vi "扫频仪设计.vi"() -> ()   [LabVIEW 2018]
uses:
  <vilib>/Analysis/3filter.llb/Filter Structure Type.ctl
  <vilib>/measure/macond.llb/IIR Filter for N Chan.vi
  <vilib>/measure/NI_MAPro.lvlib
  <vilib>/Analysis/NI_AALBase.lvlib
panel:
  in  "停止":bool
  out "数值 2":dbl
  out "数值":dbl
  out "波形图":cluster{"频率间隔/kHz":dbl, "频率间隔/kHz":dbl, dbl[]}(graph)
  in  "IIR filter specifications":T1={"Topology"=enum."Butterworth", "Type"=enum."Lowpass", "Order"=1, "Lower Fc"=100.0, "Upper Fc"=200.0, "PB Ripple"=1.0, "SB Attenuation"=60.0} caption="IIR滤波器规范" {"PB Ripple" format="%0.2f"; "SB Attenuation" format="%0.2f"; "Lower Fc" format="%0.2p"; "Upper Fc" format="%0.2p"}
  in  "filter structure option":T2=10 caption="滤波器结构选项" items=["IIR二阶"=0, "IIR四阶"=1, "自动选择"=10]
  in  "频率间隔/kHz":dbl(slide)=5.0 min=0.1 max=5.0 scale=0.1..5.0
  in  "最大频率/kHz":dbl(slide)=10.0 min=10.0 max=200.0 scale=10.0..200.0
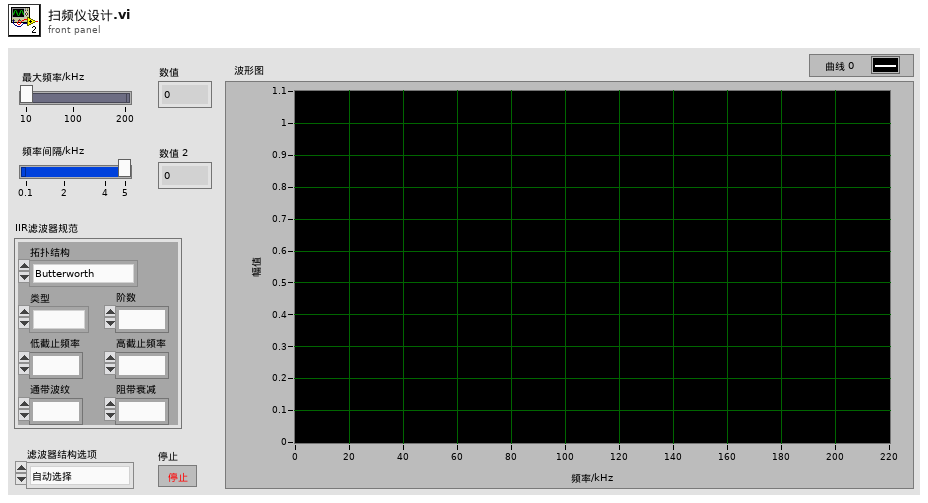
[diagram p1: front panel]
types:
  T1 = cluster{"Topology":enum16{"Off", "Butterworth", "Chebyshev", "Inverse Chebyshev", "Elliptic", "Bessel"}, "Type":enum16{"Lowpass", "Highpass", "Bandpass", "Bandstop"}, "Order":i32, "Lower Fc":dbl, "Upper Fc":dbl, "PB Ripple":dbl, "SB Attenuation":dbl}
  T2 = typedef "NI_AALBase.lvlib/Filter Structure Type.ctl" = u16
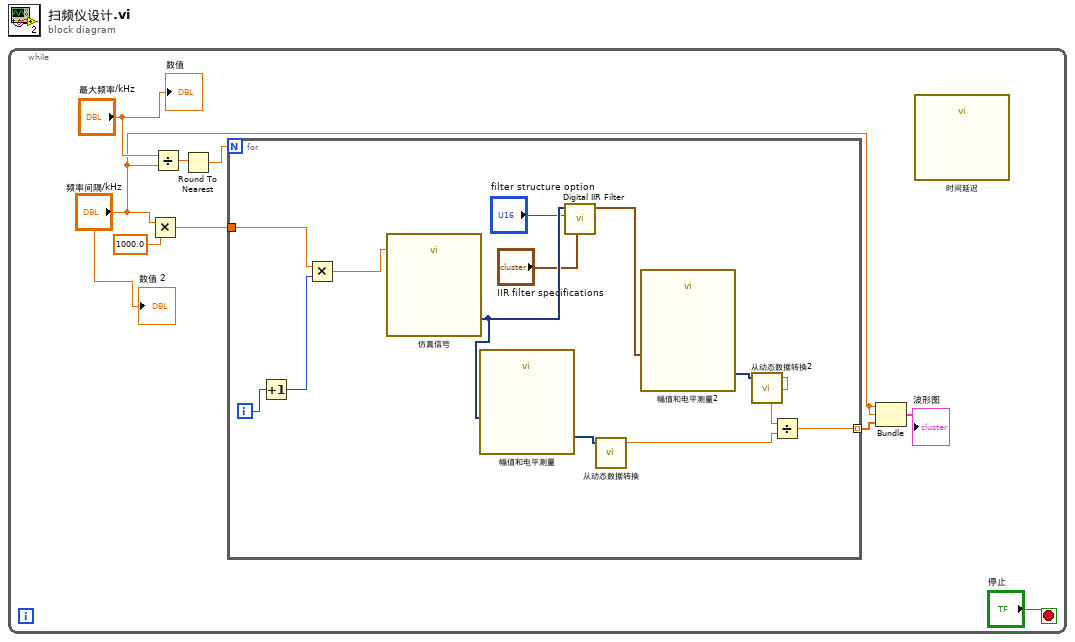
[diagram p0: block diagram]
diagram:
  n1 = while {
    stop <- "停止" stop-if-true
    n2 = Multiply(x="频率间隔/kHz", y=1000.0) -> (x*y=w6:dbl)
    n3 = Divide(x="最大频率/kHz", y="频率间隔/kHz") -> (x/y=w9:dbl)
    n4 = Round To Nearest(number=w9) -> (nearest integer value=w8:dbl)
    n5 = for {
      N: w8 -> [_]
      tunnel: w6 -> [w20]
      tunnel: [w10] -> w4 mode=indexing
      i -> [w22]
      n6 = Increment(x=w22) -> (x+1=w21:i32)
      n7 = Multiply(x=w20, y=w21) -> (x*y=w19:dbl)
      n8 = call "仿真信号"("Frequency"=w19) -> ("正弦"=w17:dynamicdata)  [unwired: 13 in, 1 out]
      n9 = call "幅值和电平测量"("Signals"=w17) -> ("Peak to Peak"=w18:dynamicdata)  [unwired: 13 in, 1 out]
      n10 = call-poly <vilib>:"Digital IIR Filter.vi"("IIR filter specifications"="IIR filter specifications", "filter structure option"="filter structure option", "signal(s) in"=w17) -> ("signal(s) out"=w14:waveform(dbl)[])  [unwired: 6 in, 2 out]
      n11 = call "从动态数据转换"("Dynamic Data Type"=w18) -> ("Scalar"=w11:dbl)  [unwired: 3 in]
      n12 = call "幅值和电平测量2"("Signals"=w14) -> ("Peak to Peak"=w13:dynamicdata)  [unwired: 13 in, 1 out]
      n13 = call "从动态数据转换2"("Dynamic Data Type"=w13) -> ("Scalar"=w12:dbl)  [unwired: 3 in]
      n14 = Divide(x=w12, y=w11) -> (x/y=w10:dbl)
    }
    n15 = Bundle("频率间隔/kHz"="频率间隔/kHz", "频率间隔/kHz"="频率间隔/kHz", w4) -> (→"波形图":cluster{"频率间隔/kHz":dbl, "频率间隔/kHz":dbl, dbl[]})  [unwired: 1 in]
    n16 = call "时间延迟"() -> ()  [unwired: 11 in, 1 out]
    "数值 2" <- "频率间隔/kHz"
    "数值" <- "最大频率/kHz"
  }
